vi "OpenFPGA_Ref.vi"(8 "error in":errorcluster, 10 "RIO HANDLER":string, 11 "Bitfile path":path) -> (0 "error out":errorcluster, 3 "Refnum out":refnum<k20>)   [LabVIEW 2025, in "Automotive Vision.lvclass"]
uses:
  Automotive Vision.lvclass
  Automotive Vision.lvclass/Automotive Vision.ctl
  <instrlib>/FlexRIO/API/Host/v1/NI FlexRIO API v1.lvlib
  <vilib>/rvi/interface/nirviCloseFPGA/nirviCloseFPGA.xnode
  <vilib>/FPGAPlugInAG/Dynamic/niLvFpga_Close_Dynamic.vi
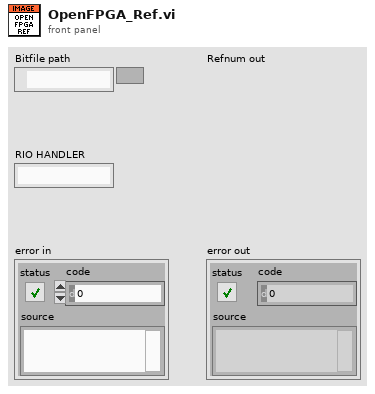
[diagram p1: front panel]
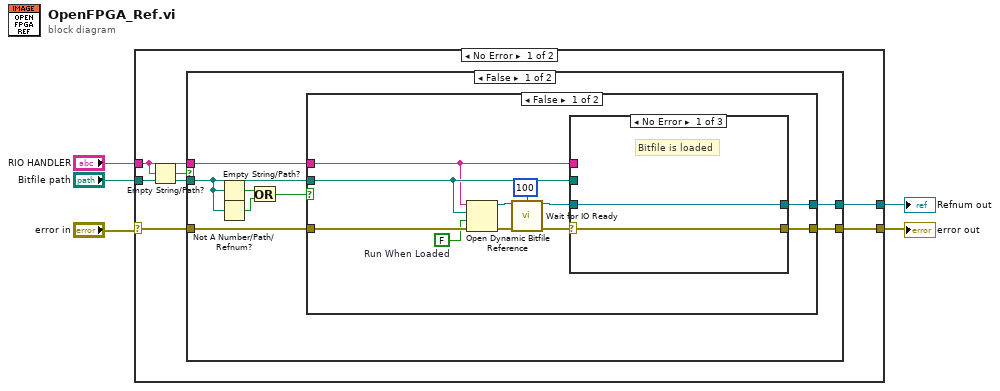
[diagram p0: block diagram]
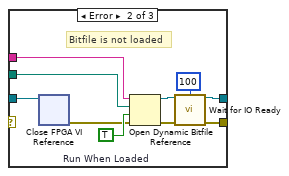
[diagram p2: hidden frame]
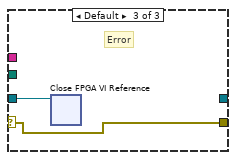
[diagram p3: hidden frame]
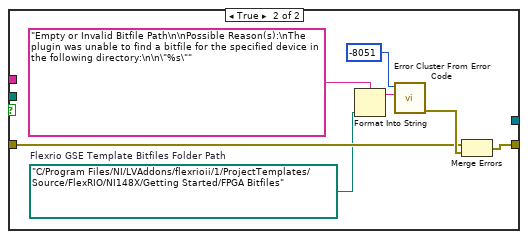
[diagram p4: hidden frame]
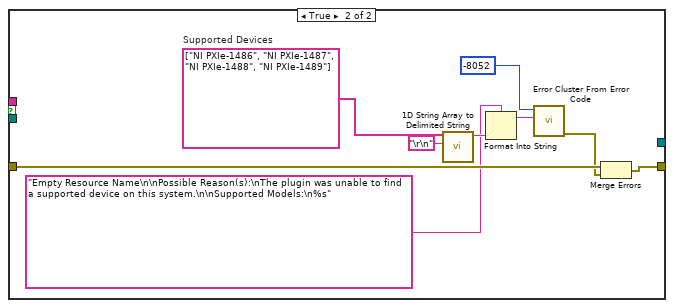
[diagram p5: hidden frame]
diagram:
  n1 = case shown="No Error" "error in" {
    selector: "error in" -> [w9 w61]
    tunnel: [w11 _] -> w2
    tunnel: [w10 w61] -> w1
    tunnel: "Bitfile path" -> [w8 _]
    tunnel: "RIO HANDLER" -> [w6 _]
    frame No Error {
      n2 = Empty String/Path?(string/path=w6) -> (empty?=w7:bool)
      n3 = case shown="False" w7 {
        tunnel: [w19 _] -> w11
        tunnel: [w18 w57] -> w10
        tunnel: w8 -> [w13 _]
        tunnel: w6 -> [w17 _]
        tunnel: w9 -> [w16 w58]
        frame False {
          n4 = Empty String/Path?(string/path=w13) -> (empty?=w14:bool)
          n5 = Not A Number/Path/Refnum?(number/path/refnum=w13) -> (NaN/Path/Refnum?=w15:bool)
          n6 = Or(x=w14, y=w15) -> (x .or. y?=w12:bool)
          n7 = case shown="False" w12 {
            tunnel: [w30 _] -> w19
            tunnel: [w29 w47] -> w18
            tunnel: w13 -> [w28 _]
            tunnel: w17 -> [w27 _]
            tunnel: w16 -> [w24 w48]
            frame False {
              w23 = FALSE  # Run When Loaded
              n8 = Open Dynamic Bitfile Reference(0:w27, 1:w28, 2:w23, 3:w24) -> (5:w21:refnum<k20>, 8:w22:errorcluster)  [unwired: 1 in]
              n9 = call <instrlib>:"Wait for IO Ready.vi"("fpga interface in"=w21, "timeout"=100, "error in"=w22) -> ("fpga interface out"=w26:refnum<k20>, "error out"=w25:errorcluster)  [unwired: 9 in, 2 out]
              n10 = case shown="No Error" w25 {
                selector: w25 -> [w32 _ w43]
                tunnel: [w32 w34 w43] -> w29
                tunnel: w26 -> [w31 w42 w44]
                tunnel: w27 -> [_ w36 _]
                tunnel: w28 -> [_ w35 _]
                tunnel: [w31 w33 _] -> w30
                frame No Error {
                  # "Bitfile is loaded"
                }
                frame Error {
                  w38 = TRUE  # Run When Loaded
                  # "Bitfile is not loaded"
                  n11 = xnode ("Close FPGA VI Reference")("FPGA VI Reference In"=w42) -> ("error out"=w37:errorcluster)  [unwired: 1 in]
                  n12 = Open Dynamic Bitfile Reference(0:w36, 1:w35, 2:w38, 3:w37) -> (5:w40:refnum<k20>, 8:w39:errorcluster)  [unwired: 1 in]
                  n13 = call <instrlib>:"Wait for IO Ready.vi"("fpga interface in"=w40, "timeout"=100, "error in"=w39) -> ("fpga interface out"=w33:refnum<k20>, "error out"=w34:errorcluster)  [unwired: 9 in, 2 out]
                }
                frame Default {
                  # "Error"
                  n14 = xnode ("Close FPGA VI Reference")("FPGA VI Reference In"=w44) -> ()  [unwired: 1 in, 1 out]
                }
              }
            }
            frame True {
              w46 = path "C:/Program Files/NI/LVAddons/flexrioii/1/ProjectTemplates/Source/FlexRIO/NI148X/Getting Started/FPGA Bitfiles"  # Flexrio GSE Template Bitfiles Folder Path
              n15 = Format Into String(format string="Empty or Invalid Bitfile Path\n\nPossible Reason(s):\nThe plugin was unable to find a bitfile for the specified device in the following directory:\n\n\"%s\"" ("-8051"), w46) -> (resulting string=w51:string)  [unwired: 2 in, 1 out]
              n16 = call <vilib>:"Error Cluster From Error Code.vi"("error message (\"\")"=w51, "error code (0)"=-8051) -> ("error out"=w49:errorcluster)  [unwired: 7 in]
              n17 = Merge Errors(w48, w49) -> (w47:errorcluster)
            }
          }
        }
        frame True {
          w54 = string[] ["NI PXIe-1486", "NI PXIe-1487", "NI PXIe-1488", "NI PXIe-1489"]  # Supported Devices
          n18 = call <vilib>:"1D String Array to Delimited String.vi"("delimiter"="\r\n", "string array"=w54) -> ("delimited string"=w53:string)  [unwired: 9 in]
          n19 = Format Into String(format string="Empty Resource Name\n\nPossible Reason(s):\nThe plugin was unable to find a supported device on this system.\n\nSupported Models:\n%s" ("-8052"), w53) -> (resulting string=w60:string)  [unwired: 2 in, 1 out]
          n20 = call <vilib>:"Error Cluster From Error Code.vi"("error message (\"\")"=w60, "error code (0)"=-8052) -> ("error out"=w56:errorcluster)  [unwired: 7 in]
          n21 = Merge Errors(w58, w56) -> (w57:errorcluster)
        }
      }
    }
    frame Error {
    }
  }
  "error out" <- w1
  "Refnum out" <- w2
